vi "LWXPS_HardwareDateAndTimeSet.vi"(6 "LabVIEW error IN":errorcluster, 8 "Date And Time":string, 9 "XPS Reference IN":refnum<k24>) -> (0 "LabVIEW error OUT":errorcluster, 1 "XPS Error String":string, 2 "Returned error code":i32, 3 "XPS Reference OUT":refnum<k24>)   [LabVIEW 2014]
uses:
  D:/XPSQ8_LabView_Library/Development/Source/Dll/Newport.XPS.CommandInterface.dll
  Dll/Newport.XPS.CommandInterface.dll
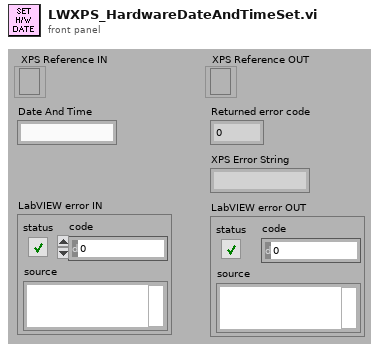
[diagram p1: front panel]
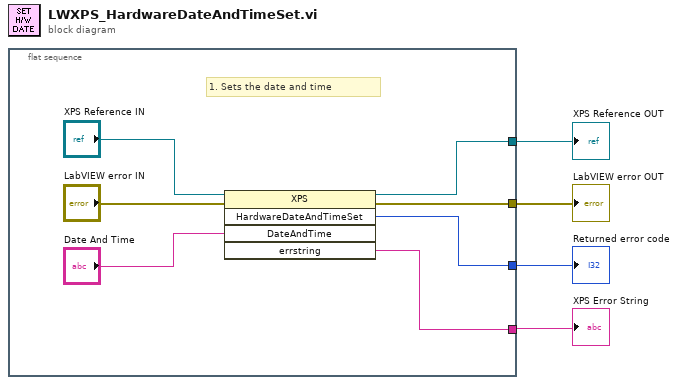
[diagram p0: block diagram]
diagram:
  n1 = flat-sequence {
    tunnel: [w5] -> w4
    tunnel: [w9] -> w3
    tunnel: [w10] -> w2
    tunnel: [w7] -> w1
    frame #0 {
      # "1. Sets the date and time"
      n2 = invoke class="XPS" method="HardwareDateAndTimeSet"(reference="XPS Reference IN", error in="LabVIEW error IN", "DateAndTime"="Date And Time") -> (reference out=w5:refnum<k24>, error out=w9:errorcluster, "HardwareDateAndTimeSet"=w10:i32, "errstring"=w7:string)  [unwired: 2 in, 1 out]
    }
  }
  "XPS Reference OUT" <- w4
  "LabVIEW error OUT" <- w3
  "Returned error code" <- w2
  "XPS Error String" <- w1
